vi "Write Channel to TDMS Log File.vi"(6 "Data":dbl[](array[numeric]), 8 "error in (no error)":errorcluster, 9 "Channel Name in":string, 10 "Group Name in":string, 11 "TDMS Log File in":refnum<class "TDMS Log File.lvclass">) -> (0 "error out":errorcluster, 3 "TDMS Log File out":refnum<class "TDMS Log File.lvclass">)   [LabVIEW 2015, in "Waveform Data Logger Engine.lvlib" / "TDMS Log File.lvclass"]
uses:
  TDMS Log File.lvclass
  TDMS Log File.lvclass/TDMS Log File.ctl
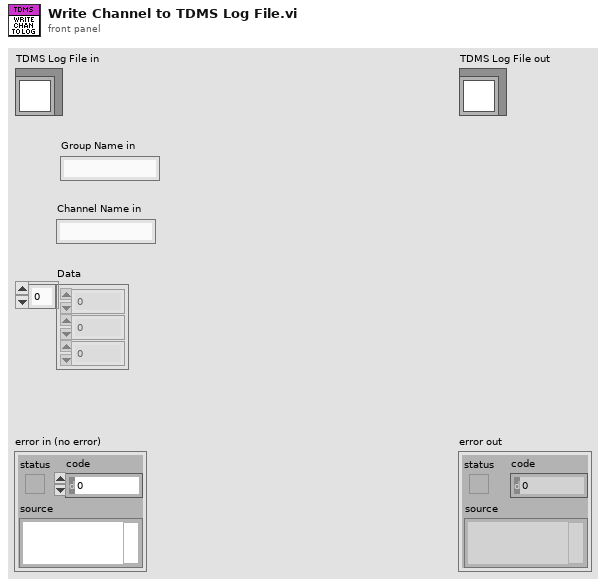
[diagram p1: front panel]
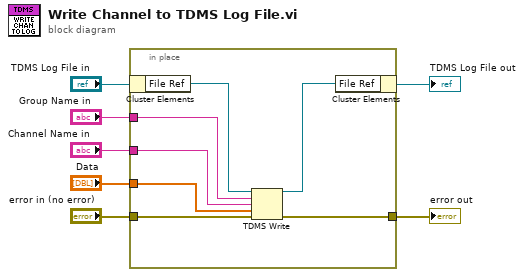
[diagram p0: block diagram]
diagram:
  n1 = in-place {
    in-place-border: "error in (no error)" -> [w14]
    in-place-border: [w12] -> w5
    in-place-border: "Data" -> [w8]
    in-place-border: "Group Name in" -> [w10]
    in-place-border: "Channel Name in" -> [w9]
    n2 = in-place-cluster #1("TDMS Log File in") -> ("File Ref"=w13:refnum<k34>)
    n3 = TDMS Write(0:w13, 5:w10, 7:w9, 9:w8, 11:w14) -> (4:w11:refnum<k34>, 15:w12:errorcluster)  [unwired: 1 in, 2 out]
    n4 = in-place-cluster #1("File Ref"=w11) -> (→"TDMS Log File out":refnum<class "TDMS Log File.lvclass">)
  }
  "error out" <- w5
